vi "Set Device and Channel IDs in IO Node.vi"(8 "error in (no error)":errorcluster, 9 "Device Number":i32, 10 "Bus Number":i32, 11 "Panel in":refnum<vi>) -> (0 "error out":errorcluster)   [LabVIEW 2014, in "SPI Engine Scripting.lvlib"]
doc: "Changes two values in the Command control on the front panel of the new IO Node: Device ID and Channel (Node) ID."
uses:
  SPI Engine Scripting.lvlib
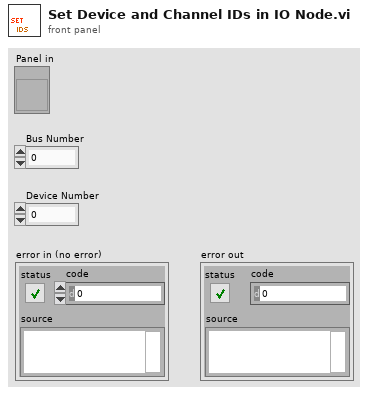
[diagram p1: front panel]
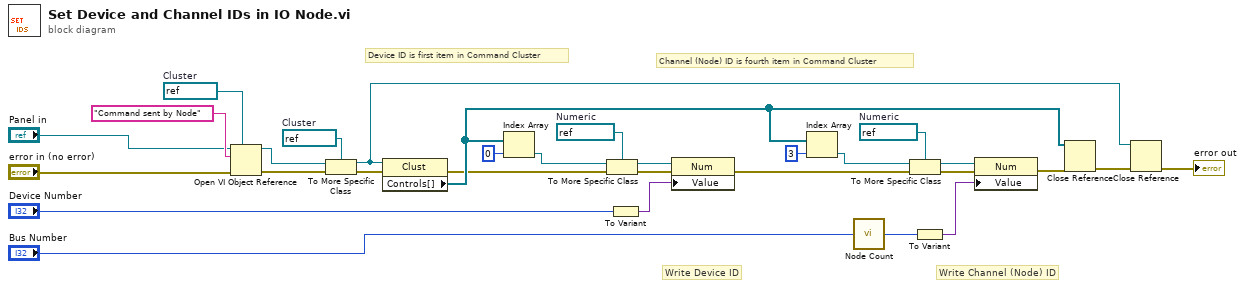
[diagram p0: block diagram]
diagram:
  w21 = refnum<vi> refnum  # Numeric
  w10 = refnum<vi> refnum  # Numeric
  w7 = refnum<vi> refnum  # Cluster
  w8 = refnum<vi> refnum  # Cluster
  # "Channel (Node) ID is fourth item in Command Cluster"
  # "Write Channel (Node) ID"
  # "Device ID is first item in Command Cluster"
  # "Write Device ID"
  n1 = Open VI Object Reference(7:w8, 8:"error in (no error)", 10:"Command sent by Node" ("name/order"), 11:"Panel in") -> (0:w5:errorcluster, 3:w4:refnum<vi>)
  n2 = To More Specific Class(target class=w7, reference=w4, error in=w5) -> (specific class reference=w9:refnum<vi>, error out=w6:errorcluster)
  n3 = property class="Clust"(reference=w9, error in=w6) -> (error out=w2:errorcluster, "Controls[]"=w27:refnum<vi>[])  [unwired: 1 out]
  n4 = Index Array(array=w27, index=0) -> (element=w12:refnum<vi>)
  n5 = To More Specific Class(target class=w10, reference=w12, error in=w2) -> (specific class reference=w13:refnum<vi>, error out=w14:errorcluster)
  n6 = To Variant(anything="Device Number") -> (Variant=w15:variant)
  n7 = property class="Num"(reference=w13, error in=w14, "Value"=w15) -> (error out=w22:errorcluster)  [unwired: 1 out]
  n8 = Index Array(array=w27, index=3) -> (element=w19:refnum<vi>)
  n9 = call "Node Count.vi"("Bus Number in"="Bus Number") -> ("Node Number"=w24:i32)
  n10 = To More Specific Class(target class=w21, reference=w19, error in=w22) -> (specific class reference=w18:refnum<vi>, error out=w17:errorcluster)
  n11 = To Variant(anything=w24) -> (Variant=w16:variant)
  n12 = property class="Num"(reference=w18, error in=w17, "Value"=w16) -> (error out=w28:errorcluster)  [unwired: 1 out]
  n13 = Close Reference(reference=w27, error in (no error)=w28) -> (error out=w26:errorcluster)
  n14 = Close Reference(reference=w9, error in (no error)=w26) -> (error out=→"error out":errorcluster)
